vi "motor数据解析.vi"(11 "字符串":string) -> (3 "扭矩":dbl format="%#_10f")   [LabVIEW 2017]
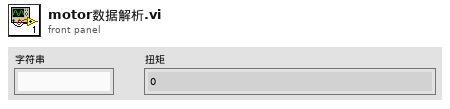
[diagram p1: front panel]
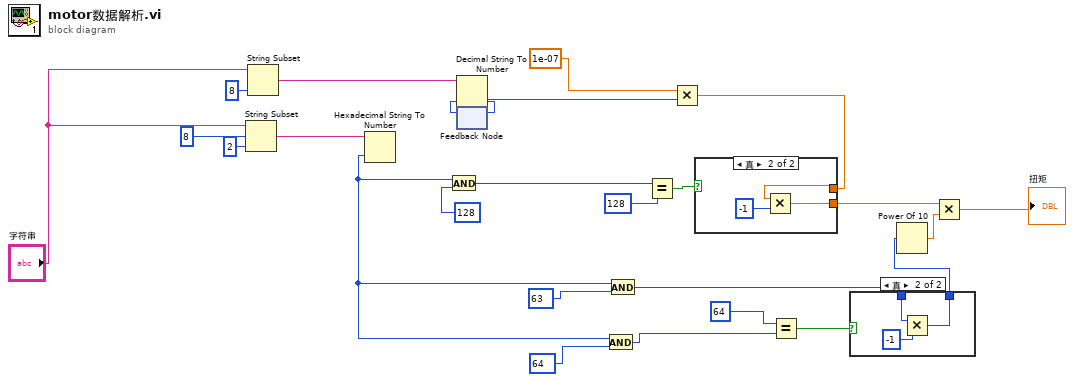
[diagram p0: block diagram]
diagram:
  n1 = String Subset(string="字符串", offset (0)=8 ("偏移量(0)"), length (rest)=2 ("长度（剩余）")) -> (substring=w25:string)
  n2 = String Subset(string="字符串", length (rest)=8 ("长度（剩余）")) -> (substring=w5:string)  [unwired: 1 in]
  n3 = Hexadecimal String To Number(string=w25) -> (number=w19:u32)  [unwired: 2 in, 1 out]
  n4 = And(x=w19, y=128) -> (x .and. y?=w11:u32)
  n5 = feedback #1() -> (w1:i32)  [unwired: 1 in]
  n6 = Decimal String To Number(string=w5, default (0L)=w1) -> (number=w2:i32)  [unwired: 1 in, 1 out]
  n7 = feedback-in #1(w2) -> ()
  n8 = And(x=w19, y=64) -> (x .and. y?=w17:u32)
  n9 = And(x=w19, y=63) -> (x .and. y?=w21:u32)
  n10 = Equal?(x=w11, y=u32 128) -> (x = y?=w15:bool)
  n11 = Multiply(x=1e-07, y=w2) -> (x*y=w23:dbl)
  n12 = case shown="真" w15 {
    tunnel: w23 -> [w26 w28]
    tunnel: [w26 w27] -> w13
    frame False {
    }
    frame True {
      n13 = Multiply(x=w28, y=-1) -> (x*y=w27:dbl)
    }
  }
  n14 = Equal?(x=u32 64, y=w17) -> (x = y?=w22:bool)
  n15 = case shown="真" w22 {
    tunnel: w21 -> [w30 w32]
    tunnel: [w30 w31] -> w24
    frame False {
    }
    frame True {
      n16 = Multiply(x=w32, y=-1) -> (x*y=w31:u32)
    }
  }
  n17 = Power Of 10(x=w24) -> (10^x=w12:dbl)
  n18 = Multiply(x=w13, y=w12) -> (x*y=→"扭矩":dbl)
